vi "GrabCallBackThread2.vi"(11 "Error IN":errorcluster) -> (15 "Error OUT":errorcluster)   [LabVIEW 2014]
uses:
  <vilib>/addons/PixeLINK/Low Level Functions/TRANSLATION.llb/TDPU-Translation-CallBackFlags.ctl
  <vilib>/addons/PixeLINK/Low Level Functions/TRANSLATION.llb/TDPU-Translation-CallbacksInfo.ctl
  <vilib>/addons/PixeLINK/Low Level Functions/ACQUISITION.llb/TDPU-Acquisition-Frame_Desc.ctl
  <vilib>/addons/PixeLINK/Low Level Functions/TRANSLATION.llb/TDPU-Translation-PixelFormat.ctl
  <vilib>/addons/PixeLINK/Low Level Functions/ACQUISITION.llb/TDPU-Acquisition-StreamState.ctl
  <vilib>/addons/PixeLINK/Low Level Functions/CAMERA_FEATURES.llb/TDPU-CameraFeatures-FeatureIds.ctl
  <vilib>/addons/PixeLINK/Low Level Functions/CAMERA_FEATURES.llb/TDPU-CameraFeatures-FeatureFlags.ctl
  PxLLabVIEW.dll
panel:
  out "Loop info":string
  in  "Exposure time":dbl=7e-05 min=7e-05 max=5.0
  out "Intensity Graph":u16[][](graph)
  out "Frame Number":u32
  out "Missed Frames":u32
  out "FrameData_FORMAT":T1 items=["PIXEL_FORMAT_MONO8", "PIXEL_FORMAT_MONO16", "PIXEL_FORMAT_YUV422", "PIXEL_FORMAT_BAYER8", "PIXEL_FORMAT_BAYER16", "PIXEL_FORMAT_RGB24", "PIXEL_FORMAT_RGB48"]
  out "FRAME_DESC":T2 {"PixelAddressingMode"."fValue" format="%.2f"; "Rotate"."fValue" format="%.2f"; "WhiteShading"."fBlueGain" format="%.2f"; "WhiteShading"."fGreenGain" format="%.2f"; "WhiteShading"."fRedGain" format="%.2f"; "AutoROI"."fHeight" format="%.2f"; "AutoROI"."fWidth" format="%.2f"; "AutoROI"."fTop" format="%.2f"; "AutoROI"."fLeft" format="%.2f"; "ExtendedShutter"."fKneePoint" format="%.2f"; "PixelFormat"."fValue" format="%.2f"; "PixelAddressingValue"."fValue" format="%.2f"; "Flip"."fVertical" format="%.2f"; "Flip"."fHorizontal" format="%.2f"; "ROI"."fHeight" format="%.2f"; "ROI"."fWidth" format="%.2f"; "ROI"."fTop" format="%.2f"; "ROI"."fLeft" format="%.2f"; "FrameRate"."fValue" format="%.2f"; "GPIO"."fParameter3" format="%.2f"; "GPIO"."fParameter2" format="%.2f"; "GPIO"."fParameter1" format="%.2f"; "GPIO"."fPolarity" format="%.2f"; "GPIO"."fMode" format="%.2f"; "OpticalFilter"."fValue" format="%.2f"; "Tilt"."fValue" format="%.2f"; "Pan"."fValue" format="%.2f"; "Zoom"."fValue" format="%.2f"; "Trigger"."fParameter" format="%.2f"; "Trigger"."fDelay" format="%.2f"; "Trigger"."fPolarity" format="%.2f"; "Trigger"."fType" format="%.2f"; "Trigger"."fMode" format="%.2f"; "Temperature"."fValue" format="%.2f"; "Focus"."fValue" format="%.2f"; "Iris"."fValue" format="%.2f"; "Gain"."fValue" format="%.2f"; "Shutter"."fValue" format="%.2f"; "Gamma"."fValue" format="%.2f"; "Saturation"."fValue" format="%.2f"; "Hue"."fValue" format="%.2f"; "WhiteBalance"."fValue" format="%.2f"; "Sharpness"."fValue" format="%.2f"; "AutoExposure"."fValue" format="%.2f"; "Brightness"."fValue" format="%.2f"; "fFrameTime" format="%.2f"}
  in  "CallbacksInfo IN":T3 {"uOverlayUse" items=["OVERLAY_PREVIEW             0x01", "OVERLAY_FORMAT_IMAGE  0x02", "OVERLAY_FORMAT_CLIP     0x04", "OVERLAY_FRAME                 0x08"]}
  out "FrameData":u8[](array[numeric]) format="%.0x"
  in  "Path IN":path
  in  "hCamera IN":u32
  in  "uOverlayUse IN":T4 items=["OVERLAY_PREVIEW             0x01", "OVERLAY_FORMAT_IMAGE  0x02", "OVERLAY_FORMAT_CLIP     0x04", "OVERLAY_FRAME                 0x08"]
  in  "Occurrence IN":refnum<k4>
  in  "Stop":bool
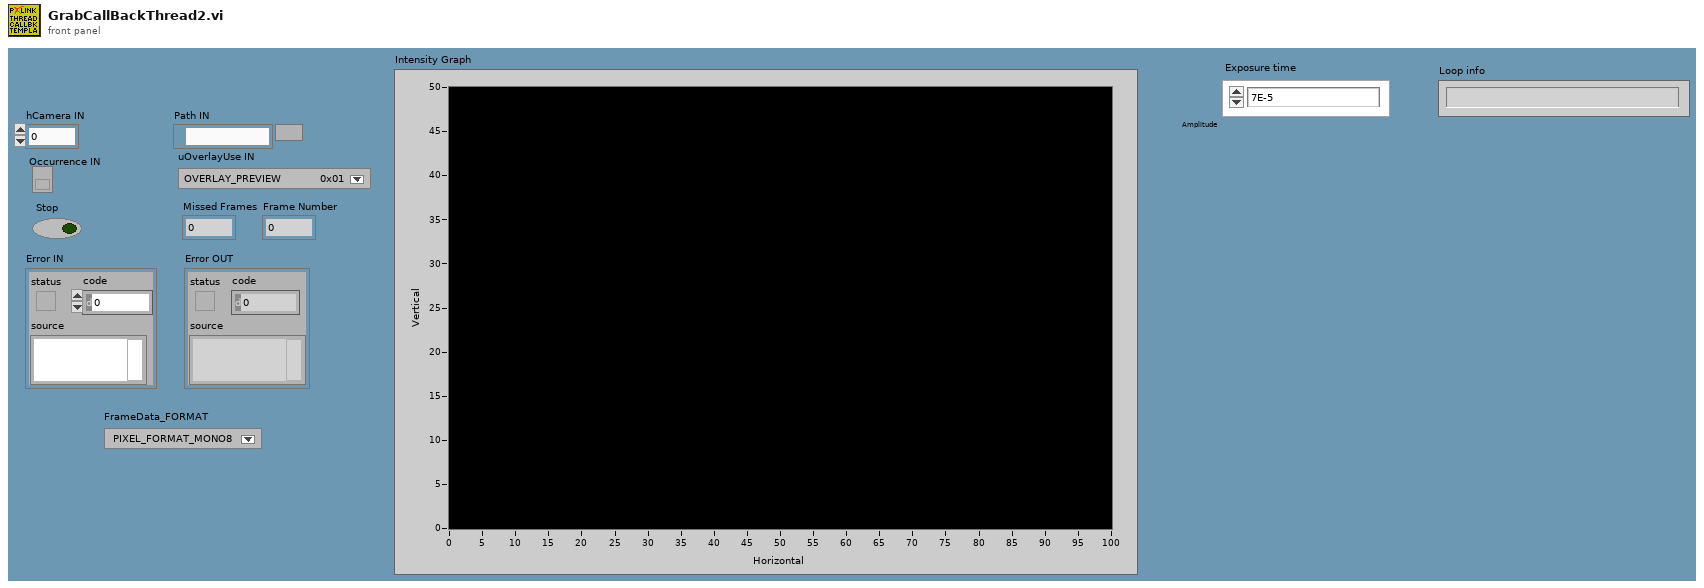
[diagram p1: front panel]
types:
  T1 = typedef "TDPU-Translation-PixelFormat.ctl" = u32
  T2 = typedef "TDPU-Acquisition-Frame_Desc.ctl" = cluster{"uSize":u32, "fFrameTime":dbl, "uFrameNumber":u32, "Brightness":cluster{"fValue":dbl}, "AutoExposure":cluster{"fValue":dbl}, "Sharpness":cluster{"fValue":dbl}, "WhiteBalance":cluster{"fValue":dbl}, "Hue":cluster{"fValue":dbl}, "Saturation":cluster{"fValue":dbl}, "Gamma":cluster{"fValue":dbl}, "Shutter":cluster{"fValue":dbl}, "Gain":cluster{"fValue":dbl}, "Iris":cluster{"fValue":dbl}, "Focus":cluster{"fValue":dbl}, "Temperature":cluster{"fValue":dbl}, "Trigger":cluster{"fMode":dbl, "fType":dbl, "fPolarity":dbl, "fDelay":dbl, "fParameter":dbl}, "Zoom":cluster{"fValue":dbl}, "Pan":cluster{"fValue":dbl}, "Tilt":cluster{"fValue":dbl}, "OpticalFilter":cluster{"fValue":dbl}, "GPIO":cluster{"fMode":dbl[], "fPolarity":dbl[], "fParameter1":dbl[], "fParameter2":dbl[], "fParameter3":dbl[]}, "FrameRate":cluster{"fValue":dbl}, "ROI":cluster{"fLeft":dbl, "fTop":dbl, "fWidth":dbl, "fHeight":dbl}, "Flip":cluster{"fHorizontal":dbl, "fVertical":dbl}, "PixelAddressingValue":cluster{"fValue":dbl}, "PixelFormat":cluster{"fValue":dbl}, "ExtendedShutter":cluster{"fKneePoint":dbl[]}, "AutoROI":cluster{"fLeft":dbl, "fTop":dbl, "fWidth":dbl, "fHeight":dbl}, "WhiteShading":cluster{"fRedGain":dbl, "fGreenGain":dbl, "fBlueGain":dbl}, "Rotate":cluster{"fValue":dbl}, "PixelAddressingMode":cluster{"fValue":dbl}}
  T3 = typedef "TDPU-Translation-CallbacksInfo.ctl" = cluster{"Occurrence":refnum<k4>, "hCamera":u32, "uOverlayUse":T4, "Path":path, "bGetClip":bool, "uNumberofFrameCaptured":u32, "error (Get Clip) ":errorcluster, "TerminationOccurence":refnum<k4>, "PDS Clip Path":path, "AVI Clip Path":path}
  T4 = typedef "TDPU-Translation-CallBackFlags.ctl" = u32
  T5 = typedef "TDPU-Acquisition-StreamState.ctl" = u32
  T6 = typedef "TDPU-CameraFeatures-FeatureFlags.ctl" = u32
  T7 = typedef "TDPU-CameraFeatures-FeatureIds.ctl" = u32
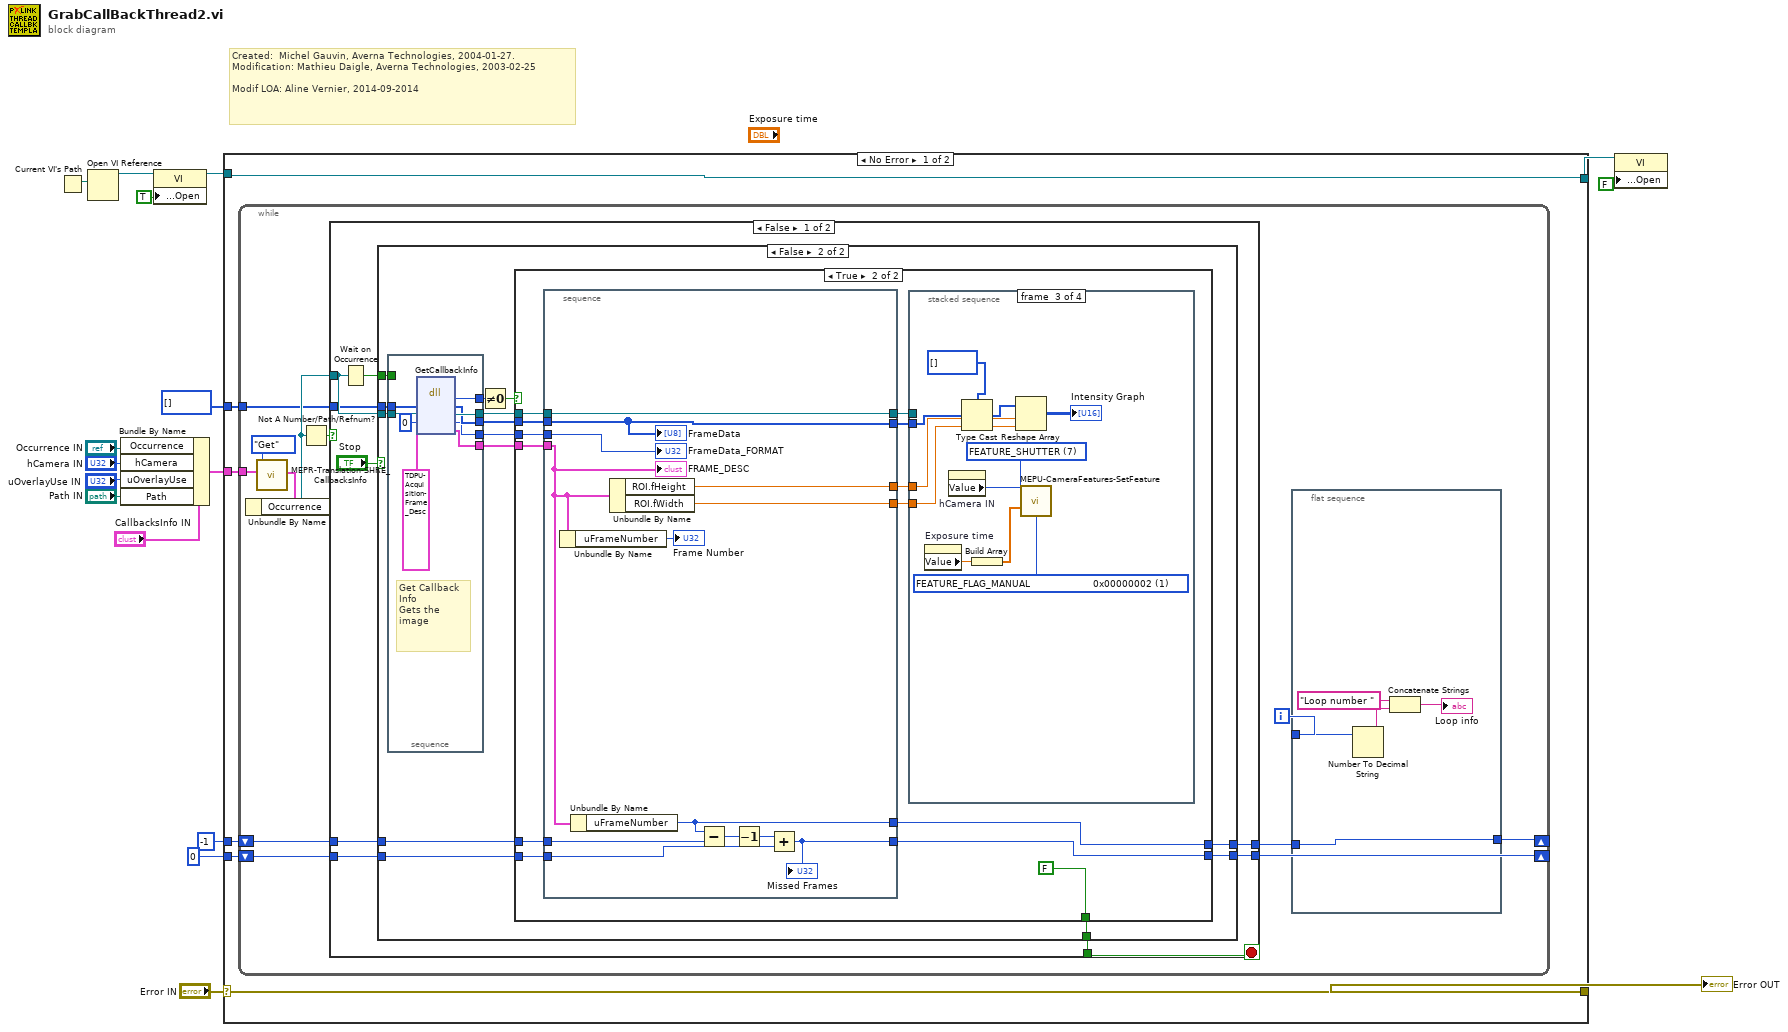
[diagram p0: block diagram]
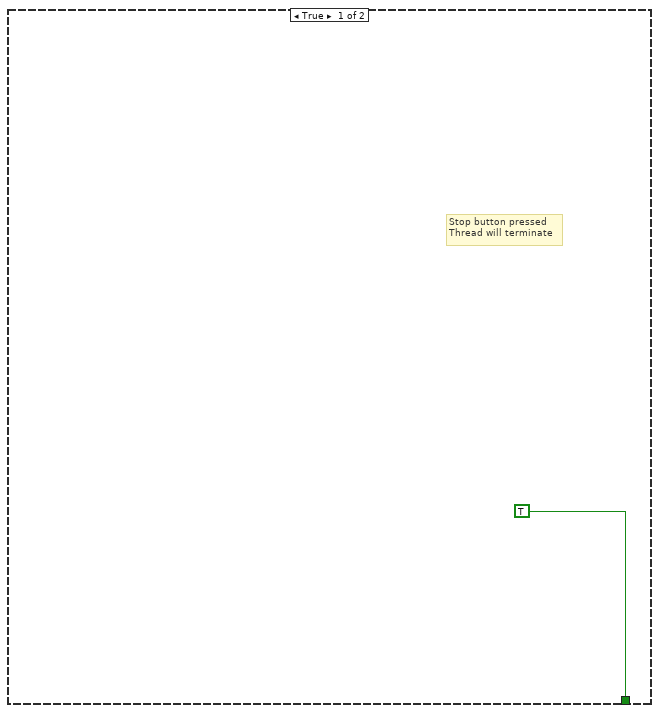
[diagram p2: hidden frame]
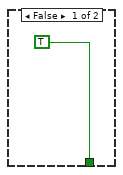
[diagram p3: hidden frame]
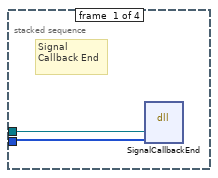
[diagram p4: hidden frame]
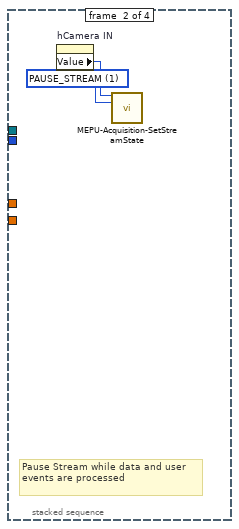
[diagram p5: hidden frame]
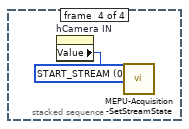
[diagram p6: hidden frame]
diagram:
  # "Created:  Michel Gauvin, Averna Technologies, 2004-01-27.\nModification: Mathieu Daigle, Averna Technologies, 2003-02-25\n\nModif LOA: Aline Vernier, 2014-09-2014"
  n1 = Current VI's Path() -> (path=w16:path)
  n2 = Open VI Reference(vi path=w16) -> (vi reference=w15:refnum<vi>)  [unwired: 5 in, 1 out]
  n3 = Bundle By Name(cluster="CallbacksInfo IN", "Occurrence"="Occurrence IN", "hCamera"="hCamera IN", "uOverlayUse"="uOverlayUse IN", "Path"="Path IN") -> (w9:T3)
  n4 = property class="VI"(reference=w15, "Front Panel Window:Open"=TRUE) -> (reference out=w13:refnum<vi>)  [unwired: 1 in, 1 out]
  n5 = case shown="No Error" "Error IN" {
    selector: "Error IN" -> [w23 w121]
    tunnel: [w23 w121] -> w17
    tunnel: w13 -> [w22 w120]
    tunnel: [w22 w120] -> w11
    tunnel: w9 -> [w21 _]
    tunnel: u8[] [] -> [w20 _]
    tunnel: u32 0 -> [w19 _]
    tunnel: -1 -> [w18 _]
    frame No Error {
      n6 = while {
        tunnel: w21 -> [w34]
        tunnel: w20 -> [w30]
        shift-right: [w25] -> _
        shift-left: w18 -> [w29]
        shift-right: [w27] -> _
        shift-left: w19 -> [w28]
        i -> [w24]
        stop <- w35 stop-if-true
        n7 = call <vilib>:"MEPR-Translation-SHRE_CallbacksInfo.vi"("Action"=enum16{"Get", "Clear", "Init", "Set"}."Get", "CallbackInfo IN"=w34) -> ("CallbackInfo OUT"=w33:T3)  [unwired: 15 in, 2 out]
        n8 = Unbundle By Name(w33) -> ("Occurrence"=w32:refnum<k4>)
        n9 = Not A Number/Path/Refnum?(number/path/refnum=w32) -> (NaN/Path/Refnum?=w36:bool)
        n10 = case shown="False" w36 {
          selector: w36 -> [_ w119]
          tunnel: w32 -> [w50 _]
          tunnel: [w42 w119] -> w35
          tunnel: w30 -> [w47 _]
          tunnel: [w46 _] -> w26
          tunnel: w29 -> [w45 _]
          tunnel: w28 -> [w44 _]
          tunnel: [w43 _] -> w27
          frame False {
            n11 = Wait on Occurrence(2:w50) -> (0:w49:bool)  [unwired: 2 in]
            n12 = case shown="False" "Stop" {
              tunnel: w50 -> [_ w65]
              tunnel: w49 -> [_ w64]
              tunnel: w47 -> [_ w61]
              tunnel: [_ w58] -> w46
              tunnel: w45 -> [_ w57]
              tunnel: w44 -> [_ w56]
              tunnel: [_ w55] -> w43
              tunnel: [TRUE w52] -> w42
              frame True {
                # "Stop button pressed\nThread will terminate"
              }
              frame False {
                n13 = stacked-sequence {
                  tunnel: w65 -> [w117]
                  tunnel: [w118] -> w53
                  tunnel: w64 -> [_]
                  tunnel: [w115] -> w63
                  tunnel: [w116] -> w62
                  tunnel: w61 -> [w114]
                  tunnel: [w111] -> w60
                  tunnel: [w110] -> w59
                  frame #0 {
                    # "Get Callback Info\nGets the image"
                    n14 = dll-call lib="PxLLabVIEW.dll" fn="GetCallbackInfo"("output param"=w114, "Occurrence"=w117, "pDataFormat"=u32 0, "FRAME_DESC"=T2 {"uSize"=0, "fFrameTime"=0.0, "uFrameNumber"=0, "Brightness"={"fValue"=0.0}, "AutoExposure"={"fValue"=0.0}, "Sharpness"={"fValue"=0.0}, "WhiteBalance"={"fValue"=0.0}, "Hue"={"fValue"=0.0}, "Saturation"={"fValue"=0.0}, "Gamma"={"fValue"=0.0}, "Shutter"={"fValue"=0.0}, "Gain"={"fValue"=0.0}, "Iris"={"fValue"=0.0}, "Focus"={"fValue"=0.0}, "Temperature"={"fValue"=0.0}, "Trigger"={"fMode"=0.0, "fType"=0.0, "fPolarity"=0.0, "fDelay"=0.0, "fParameter"=0.0}, "Zoom"={"fValue"=0.0}, "Pan"={"fValue"=0.0}, "Tilt"={"fValue"=0.0}, "OpticalFilter"={"fValue"=0.0}, "GPIO"={"fMode"=[], "fPolarity"=[], "fParameter1"=[], "fParameter2"=[], "fParameter3"=[]}, "FrameRate"={"fValue"=0.0}, "ROI"={"fLeft"=0.0, "fTop"=0.0, "fWidth"=0.0, "fHeight"=0.0}, "Flip"={"fHorizontal"=0.0, "fVertical"=0.0}, "PixelAddressingValue"={"fValue"=0.0}, "PixelFormat"={"fValue"=0.0}, "ExtendedShutter"={"fKneePoint"=[]}, "AutoROI"={"fLeft"=0.0, "fTop"=0.0, "fWidth"=0.0, "fHeight"=0.0}, "WhiteShading"={"fRedGain"=0.0, "fGreenGain"=0.0, "fBlueGain"=0.0}, "Rotate"={"fValue"=0.0}, "PixelAddressingMode"={"fValue"=0.0}}) -> (w118:i32, "output param"=w115:u8[], "Occurrence"=w116:refnum<k4>, "pDataFormat"=w110:u32, "FRAME_DESC"=w111:T2)  [unwired: 3 in, 2 out]
                  }
                }
                n15 = Not Equal To 0?(x=w53) -> (x != 0?=w54:bool)
                n16 = case shown="True" w54 {
                  tunnel: w63 -> [_ w78]
                  tunnel: w62 -> [_ w77]
                  tunnel: w60 -> [_ w76]
                  tunnel: w59 -> [_ w75]
                  tunnel: [_ w70] -> w58
                  tunnel: w57 -> [_ w74]
                  tunnel: w56 -> [_ w73]
                  tunnel: [_ w72] -> w55
                  tunnel: [TRUE FALSE] -> w52
                  frame False {
                  }
                  frame True {
                    n17 = stacked-sequence {
                      tunnel: w77 -> [w109]
                      tunnel: [w109] -> w79
                      tunnel: w78 -> [w99]
                      tunnel: w76 -> [w101]
                      tunnel: w75 -> [w102]
                      tunnel: [w108] -> w70
                      tunnel: w74 -> [w107]
                      tunnel: w73 -> [w104]
                      tunnel: [w103] -> w72
                      tunnel: [w99] -> w69
                      tunnel: [w98] -> w68
                      tunnel: [w97] -> w67
                      frame #0 {
                        n18 = Unbundle By Name(w101) -> ("uFrameNumber"=→"Frame Number":u32)
                        n19 = Unbundle By Name(w101) -> ("uFrameNumber"=w108:u32)
                        n20 = Unbundle By Name(w101) -> ("ROI.fHeight"=w98:dbl, "ROI.fWidth"=w97:dbl)
                        n21 = Subtract(x=w108, y=w107) -> (x-y=w106:u32)
                        n22 = Decrement(x=w106) -> (x-1=w105:u32)
                        n23 = Add(x=w105, y=w104) -> (x+y=w103:u32)
                        "Missed Frames" <- w103
                        "FrameData" <- w99
                        "FRAME_DESC" <- w101
                        "FrameData_FORMAT" <- w102
                      }
                    }
                    n24 = stacked-sequence {
                      tunnel: w79 -> [w81 _ _ _]
                      tunnel: w69 -> [w80 _ w93 _]
                      tunnel: w68 -> [_ _ w84 _]
                      tunnel: w67 -> [_ _ w91 _]
                      frame #0 {
                        # "Signal Callback End"
                        n25 = dll-call lib="PxLLabVIEW.dll" fn="SignalCallbackEnd"("Occurrence"=w81, "Data"=w80) -> ()  [unwired: 6 in, 2 out]
                      }
                      frame #1 {
                        w82 = T5 1 items=["START_STREAM", "PAUSE_STREAM", "STOP_STREAM"] ("uStreamState IN")
                        # "Pause Stream while data and user events are processed"
                        n26 = property on="hCamera IN" class="DigNum (strict)"() -> ("Value"=w83:u32)  [unwired: 2 in, 2 out]
                        n27 = call <vilib>:"MEPU-Acquisition-SetStreamState.vi"("hCamera IN"=w83, "uStreamState IN"=w82) -> ()  [unwired: 12 in, 2 out]
                      }
                      frame #2 {
                        w85 = T6 1 items=["FEATURE_FLAG_PRESENCE                 0x00000001", "FEATURE_FLAG_MANUAL                     0x00000002", "FEATURE_FLAG_AUTO                         0x00000004", "FEATURE_FLAG_ONEPUSH                   0x00000008", "FEATURE_FLAG_OFF                            0x00000010", "FEATURE_FLAG_DESC_SUPPORTED    0x00000020", "FEATURE_FLAG_READ_ONLY               0x00000040"] ("uFlags IN")
                        w88 = T7 7 items=["FEATURE_BRIGHTNESS", "FEATURE_EXPOSURE", "FEATURE_SHARPNESS", "FEATURE_WHITE_BAL", "FEATURE_HUE", "FEATURE_SATURATION", "FEATURE_GAMMA", "FEATURE_SHUTTER", "FEATURE_GAIN", "FEATURE_IRIS", "FEATURE_FOCUS", "FEATURE_TEMPERATURE", "FEATURE_TRIGGER", "FEATURE_ZOOM", "FEATURE_PAN", "FEATURE_TILT", "FEATURE_OPT_FILTER", "FEATURE_GPIO", "FEATURE_FRAME_RATE", "FEATURE_ROI", "FEATURE_FLIP", "FEATURE_PIXEL_ADDRESSING", "FEATURE_PIXEL_FORMAT", "FEATURE_EXTENDED_SHUTTER", "FEATURE_AUTO_ROI", "FEATURE_LOOKUP_TABLE", "FEATURE_MEMORY_CHANNEL", "FEATURE_WHITE_SHADING", "FEATURE_ROTATE", "FEATURE_IMAGER_CLK_DIVISOR", "FEATURE_TRIG_WITH_CNTRLD_LIGHT", "FEATURE_MAX_PIXEL_SIZE"] ("uFeatureId IN")
                        n28 = property on="Exposure time" class="DigNum (strict)"() -> ("Value"=w87:dbl)  [unwired: 2 in, 2 out]
                        n29 = property on="hCamera IN" class="DigNum (strict)"() -> ("Value"=w89:u32)  [unwired: 2 in, 2 out]
                        n30 = Type Cast(type=u16[] [] ("output param"), x=w93) -> (*(type *) &x=w92:u16[])
                        n31 = Build Array(w87) -> (w86:dbl[])
                        n32 = Reshape Array(w92, w84, w91) -> (→"Intensity Graph":u16[][])
                        n33 = call <vilib>:"MEPU-CameraFeatures-SetFeature.vi"("hCamera IN"=w89, "uFeatureId IN"=w88, "uFlags IN"=w85, "pParms IN"=w86) -> ()  [unwired: 9 in, 3 out]
                      }
                      frame #3 {
                        w95 = T5 0 items=["START_STREAM", "PAUSE_STREAM", "STOP_STREAM"] ("uStreamState IN")
                        n34 = property on="hCamera IN" class="DigNum (strict)"() -> ("Value"=w96:u32)  [unwired: 2 in, 2 out]
                        n35 = call <vilib>:"MEPU-Acquisition-SetStreamState.vi"("hCamera IN"=w96, "uStreamState IN"=w95) -> ()  [unwired: 12 in, 2 out]
                      }
                    }
                  }
                }
              }
            }
          }
          frame True {
          }
        }
        n36 = flat-sequence {
          tunnel: w26 -> [w41]
          tunnel: [w41] -> w25
          tunnel: w24 -> [w40]
          frame #0 {
            n37 = Number To Decimal String(number=w40) -> (decimal integer string=w38:string)  [unwired: 1 in]
            n38 = Concatenate Strings("Loop number " ("string"), w38) -> (→"Loop info":string)
          }
        }
      }
    }
    frame Error {
    }
  }
  "Error OUT" <- w17
  n39 = property class="VI"(reference=w11, "Front Panel Window:Open"=FALSE) -> ()  [unwired: 1 in, 2 out]
